vi "RFmx_Control.vi"(8 "error in (no error)":errorcluster, 10 "Device Resources":T1={"RFSG Resource in"="VST", "RFSA Resource in"="VST", "RFmx Resource in"="VST"}, 11 "Message_Queues":T2) -> (0 "error out":errorcluster)   [LabVIEW 2014]
uses:
  02_Controls/Message_Queues.ctl
  02_Controls/Message_Data_Ctl.ctl
  15_DataManagement/Device_Resources.ctl
  15_DataManagement/Config_RFmx_Settings.ctl
  <vilib>/RFmx/SpecAn/mx/RFmxSpecAn.llb/RFmxSpecAn Configure Digital Edge Trigger.vi
  <resource>/objmgr/RFmxSpecAn.rc
panel:
  out "RFSG_Msg":string
  out "Message":string
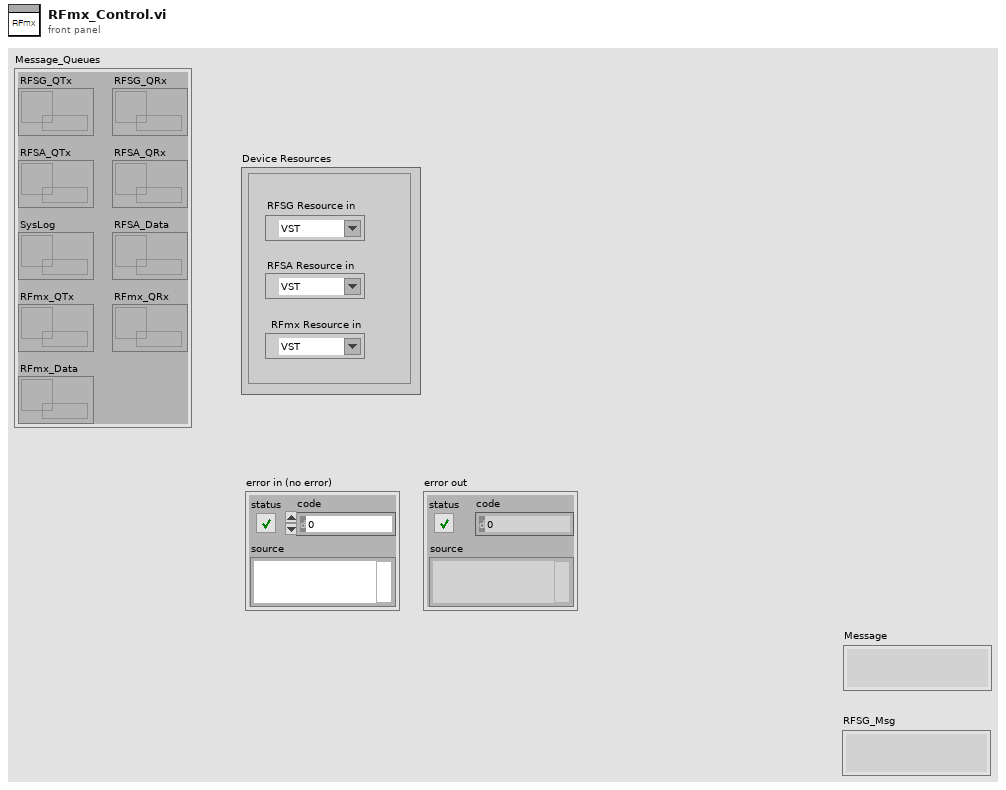
[diagram p1: front panel]
types:
  T1 = typedef "Device_Resources.ctl" = cluster{"RFSG Resource in":refnum<k15>, "RFSA Resource in":refnum<k15>, "RFmx Resource in":refnum<k15>}
  T2 = typedef "Message_Queues.ctl" = cluster{"RFSG_QTx":refnum<queue>, "RFSG_QRx":refnum<queue>, "RFSA_QTx":refnum<queue>, "RFSA_QRx":refnum<queue>, "SysLog":refnum<queue>, "RFSA_Data":refnum<queue>, "RFmx_QTx":refnum<queue>, "RFmx_QRx":refnum<queue>, "RFmx_Data":refnum<queue>}
  T3 = typedef "Config_RFmx_Settings.ctl" = cluster{"Default":cluster{"Center_Freq(Hz)":dbl, "Ref_Level(dBm)":dbl, "Span(Hz)":dbl, "RBW(Hz)":dbl, "RBW Filter Type":enum16{"FFT Based", "Gaussian", "Flat", "Synch Tuned - 4", "Synch Tuned - 5"}, "Ch_IBW(Hz)":dbl, "Sweep_Time(s)":dbl, "Num_of_Average":i32, "IQ_Bandwidth(Hz)":dbl}, "ACP_Offset_Freq":dbl[], "ACP_Offset_IBW":dbl[], "OBW_Percent(%)":dbl, "TXP_Interval(s)":dbl, "CCDF_Interval(s)":dbl, "CCDF_Threshold":dbl, "SFDR_Span(Hz)":dbl, "Harms_RBW(Hz)":dbl, "Harms_RBW_Filter":enum16{"FFT Based", "Gaussian", "Flat", "Synch Tuned - 4", "Synch Tuned - 5"}}
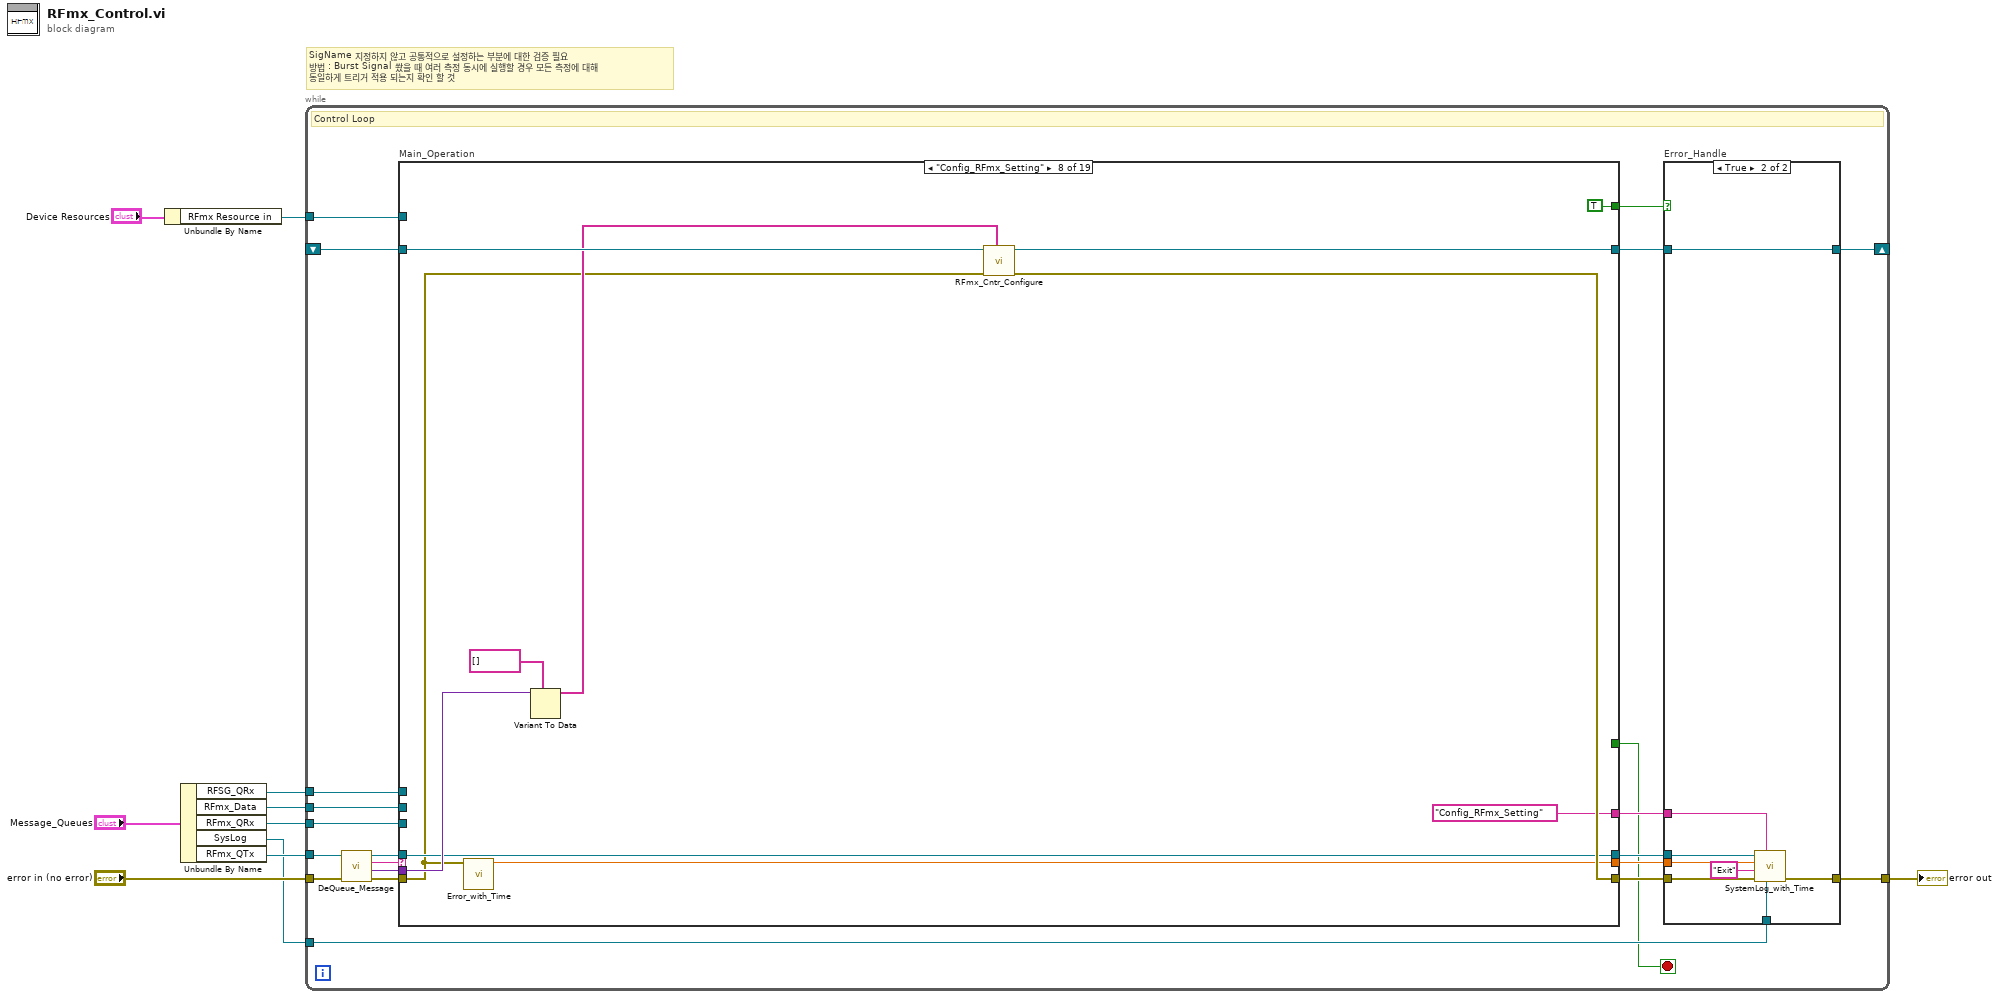
[diagram p0: block diagram]
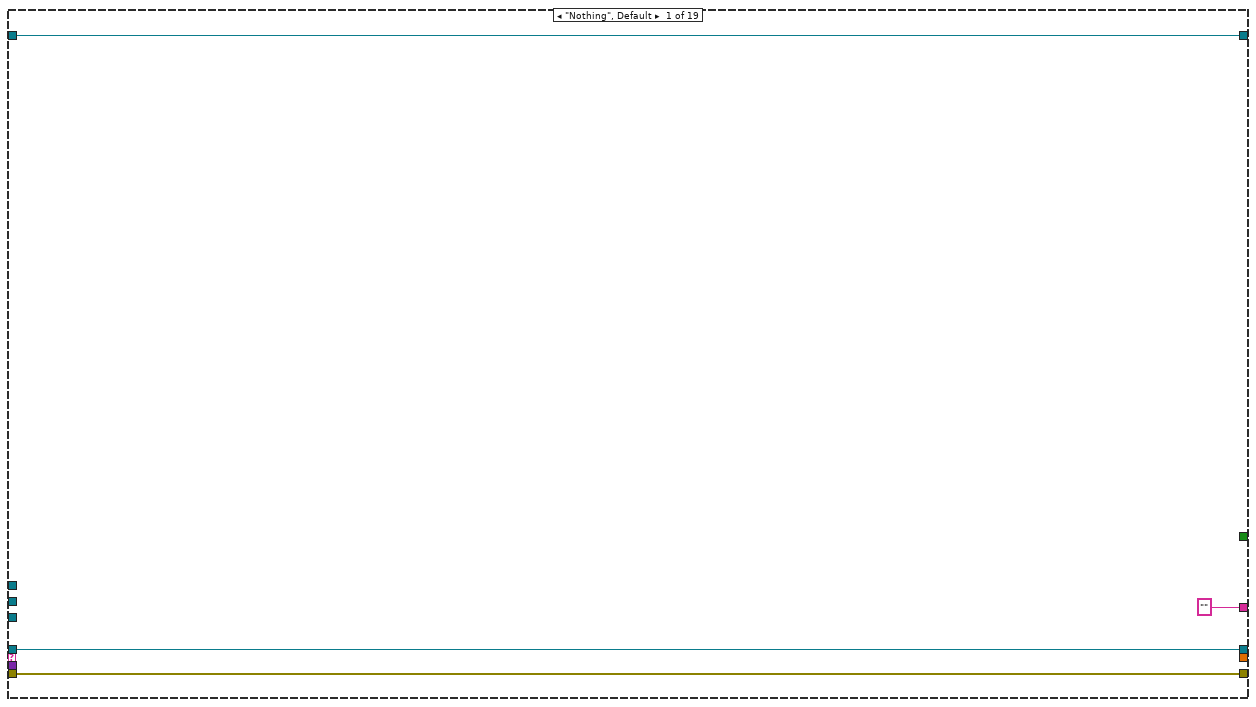
[diagram p3: hidden frame]
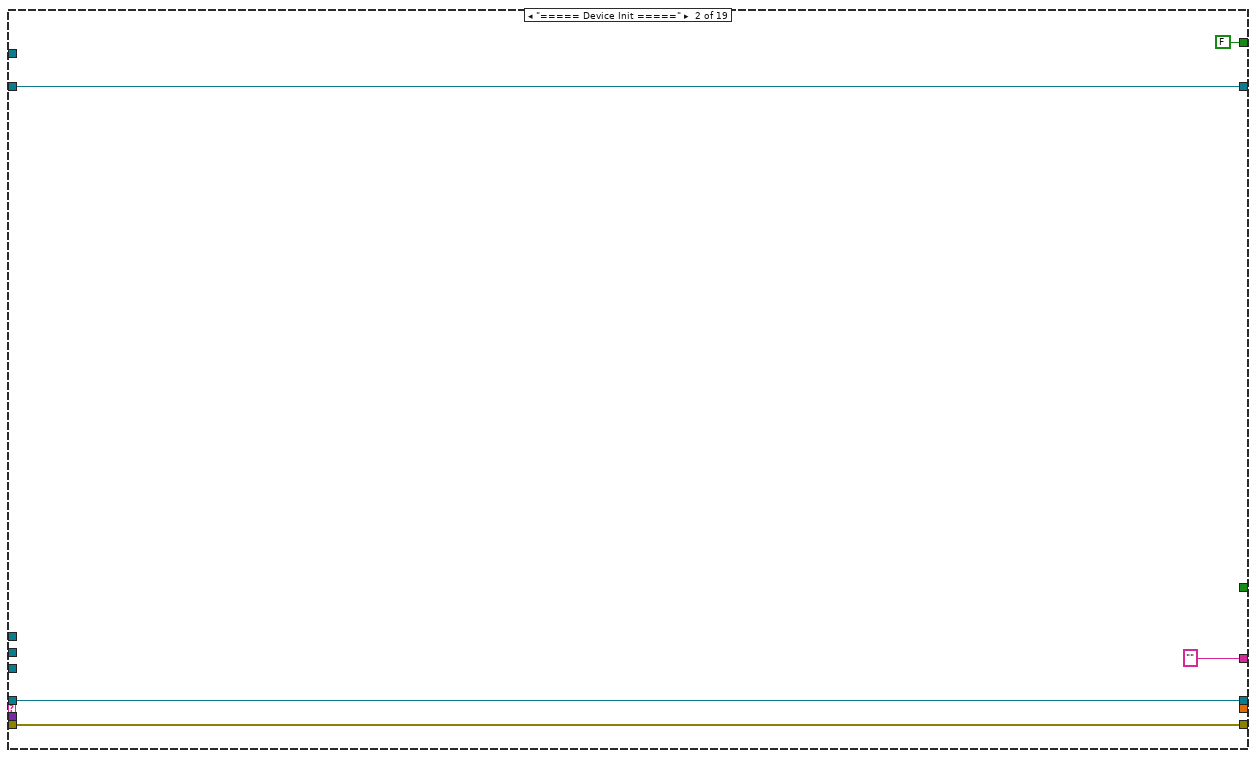
[diagram p4: hidden frame]
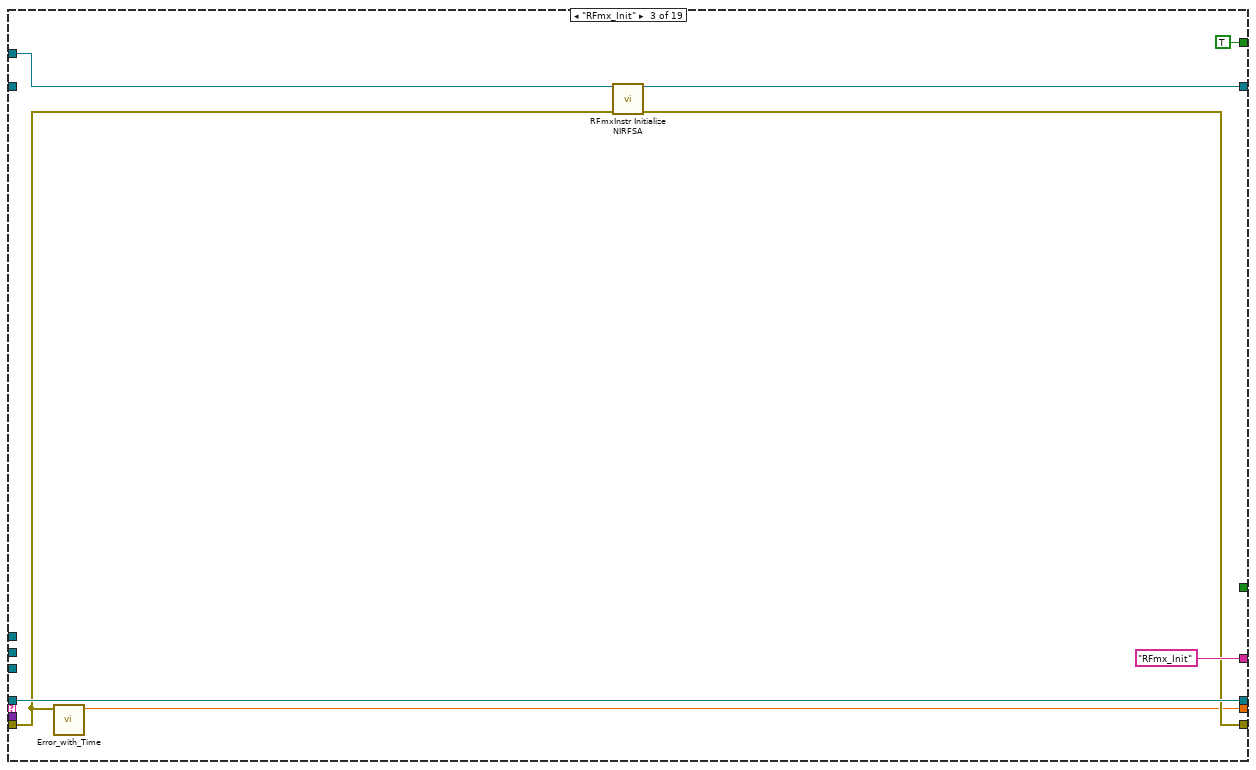
[diagram p5: hidden frame]
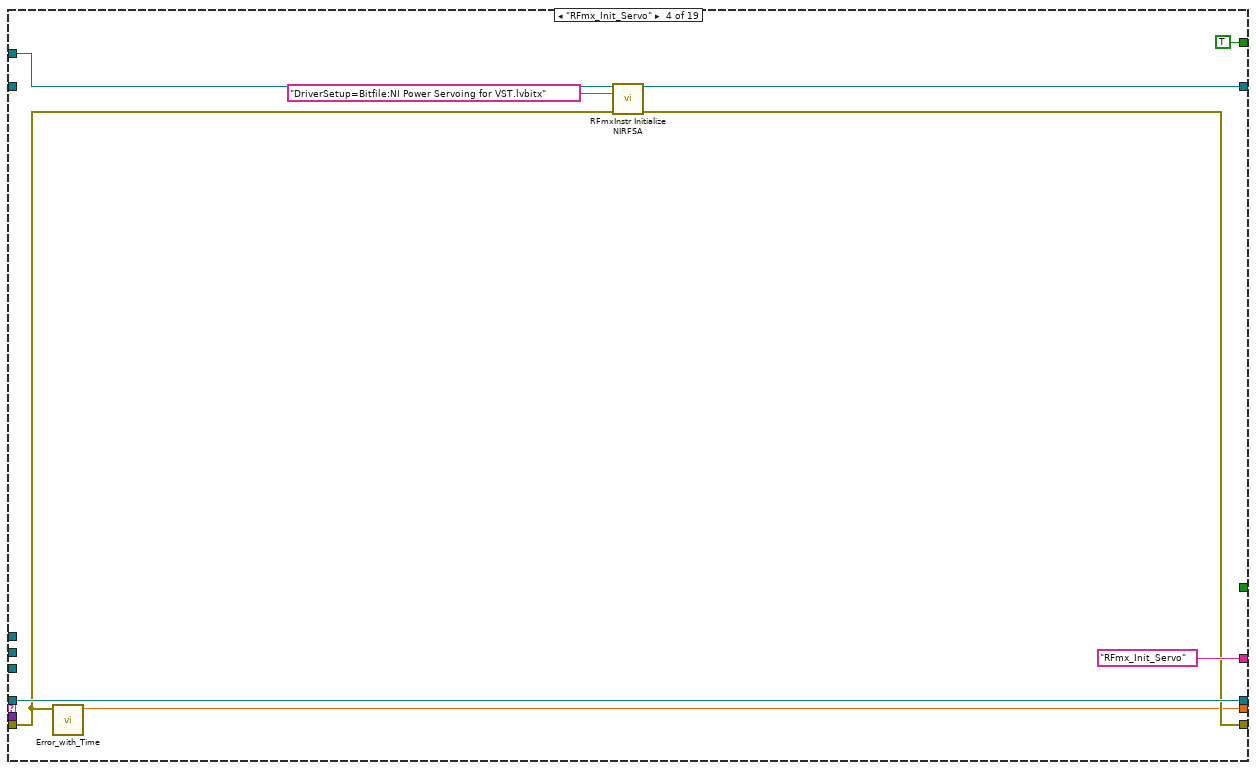
[diagram p6: hidden frame]
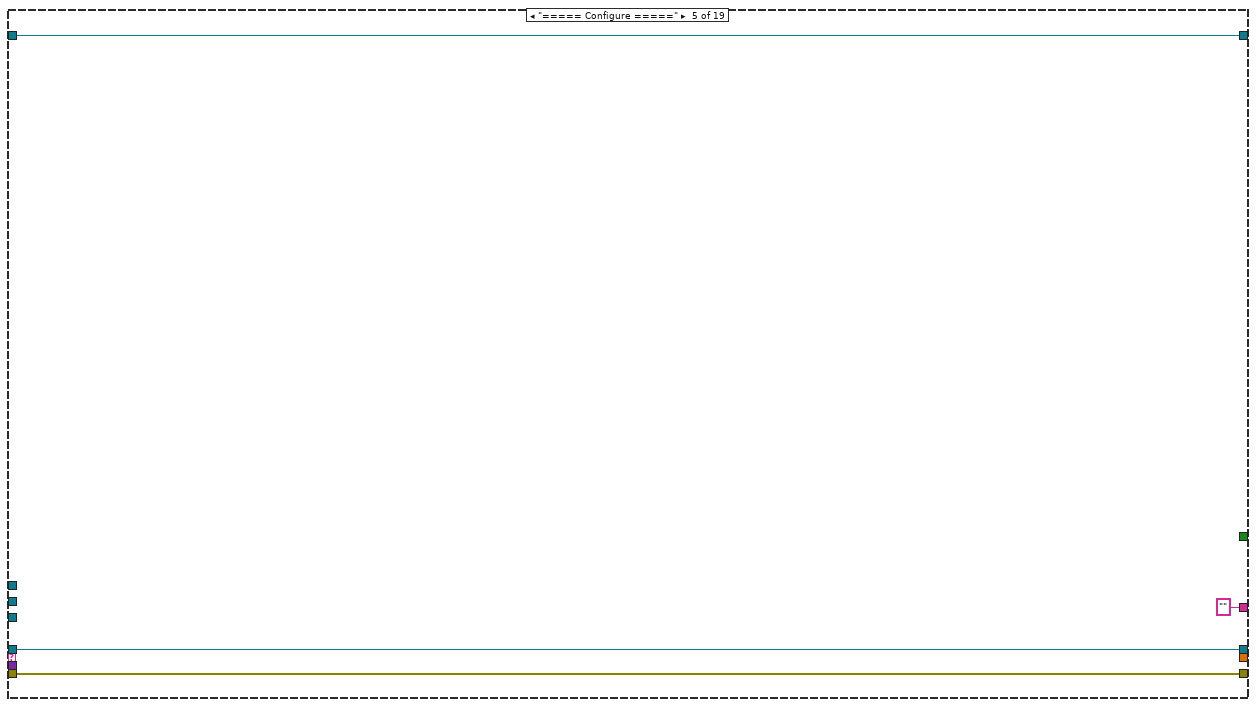
[diagram p7: hidden frame]
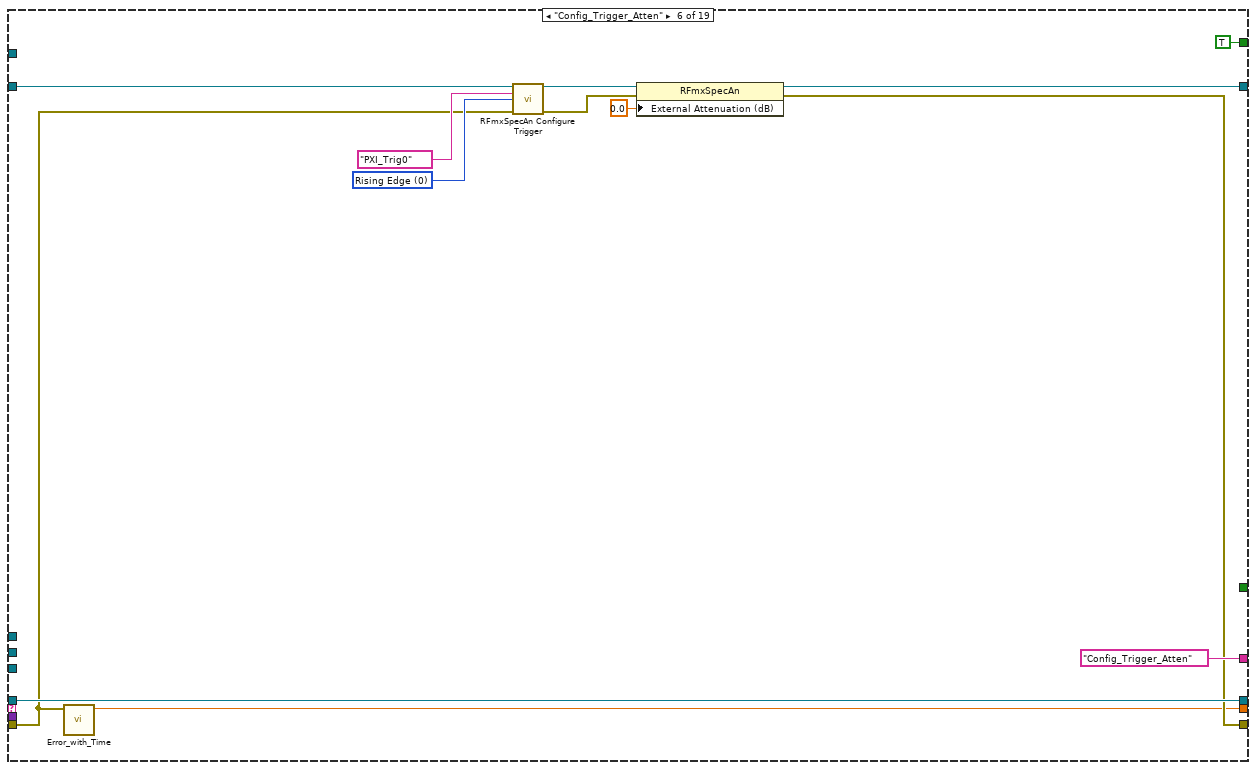
[diagram p8: hidden frame]
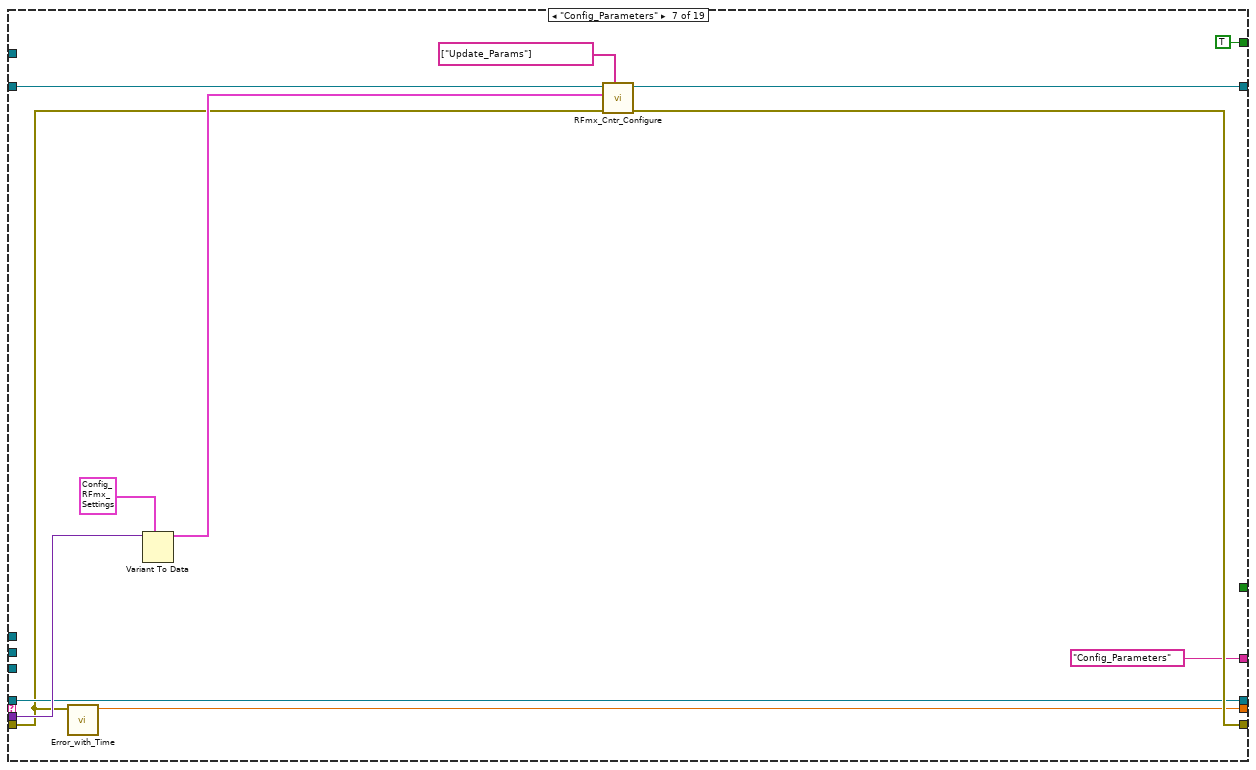
[diagram p9: hidden frame]
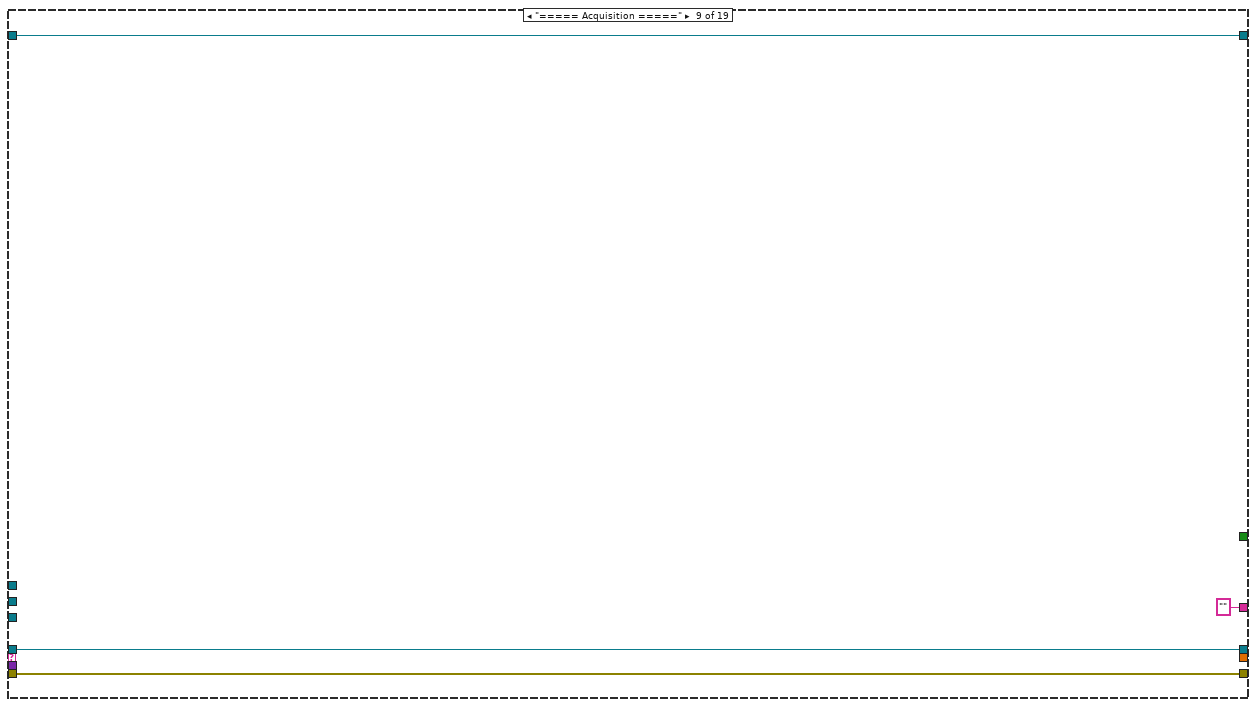
[diagram p10: hidden frame]
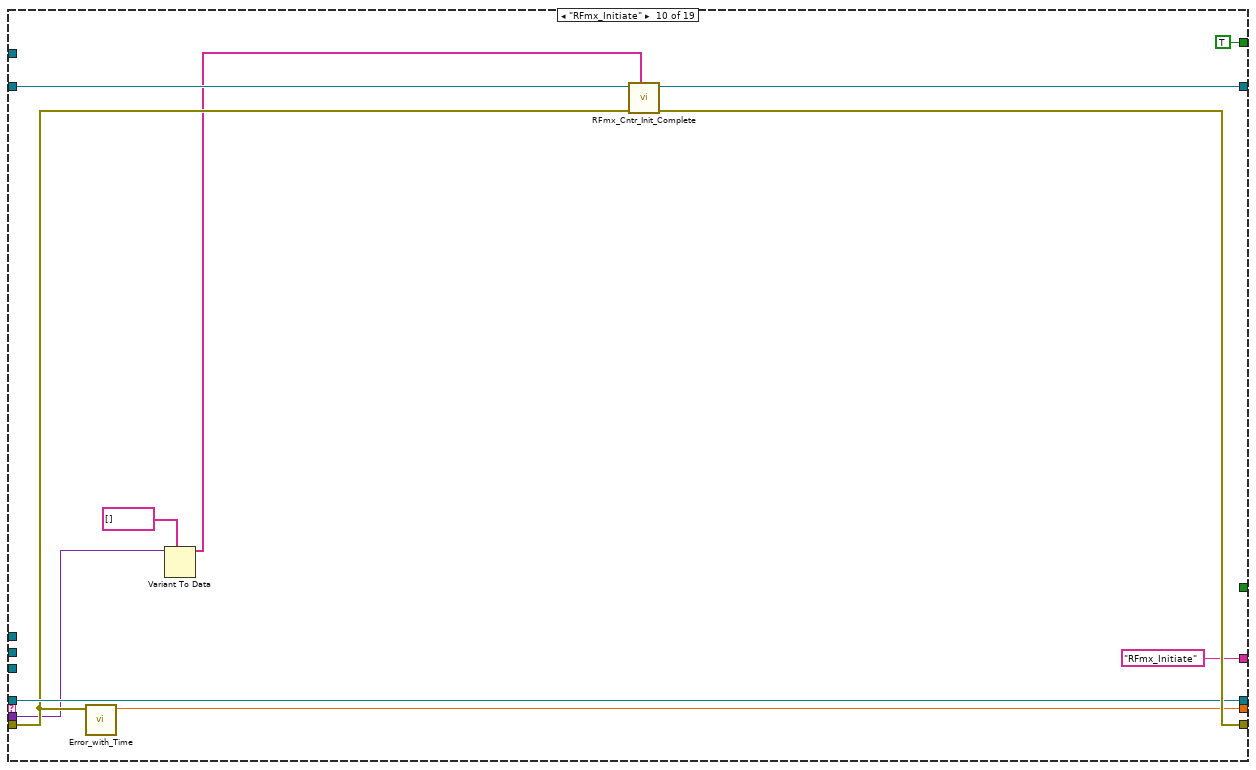
[diagram p11: hidden frame]
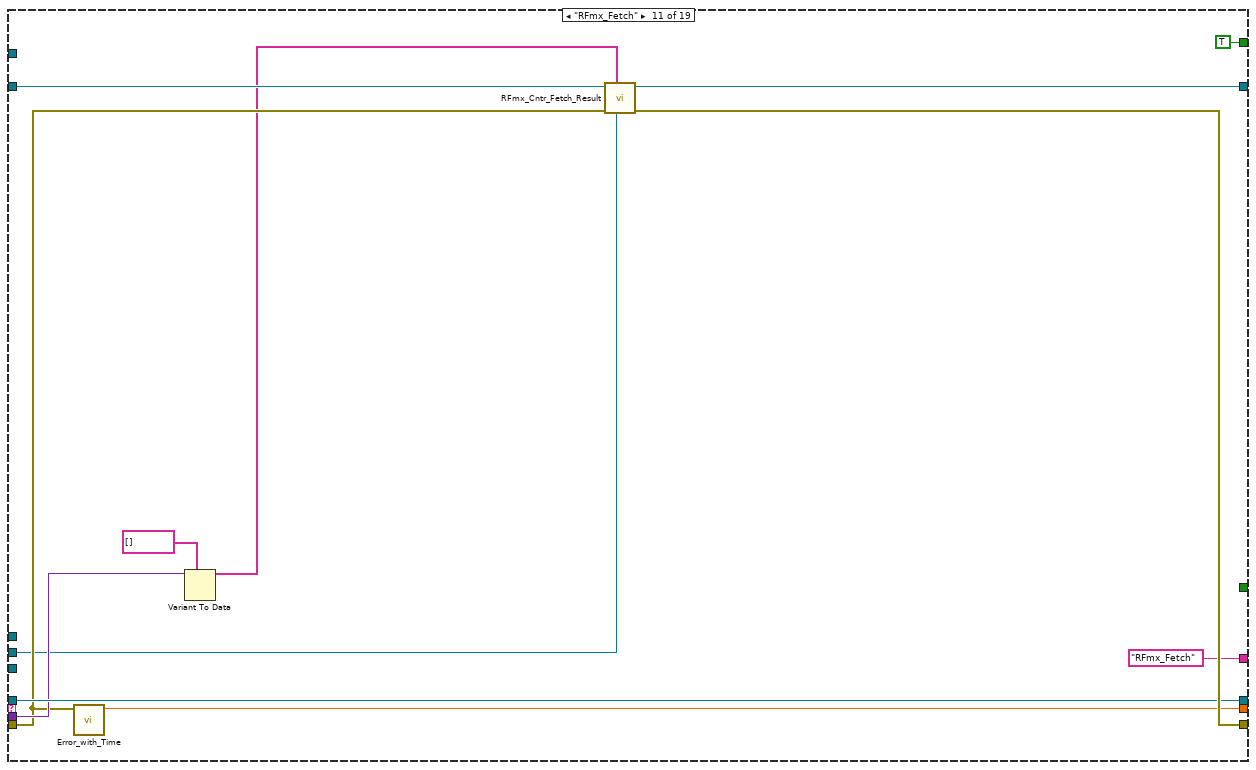
[diagram p12: hidden frame]
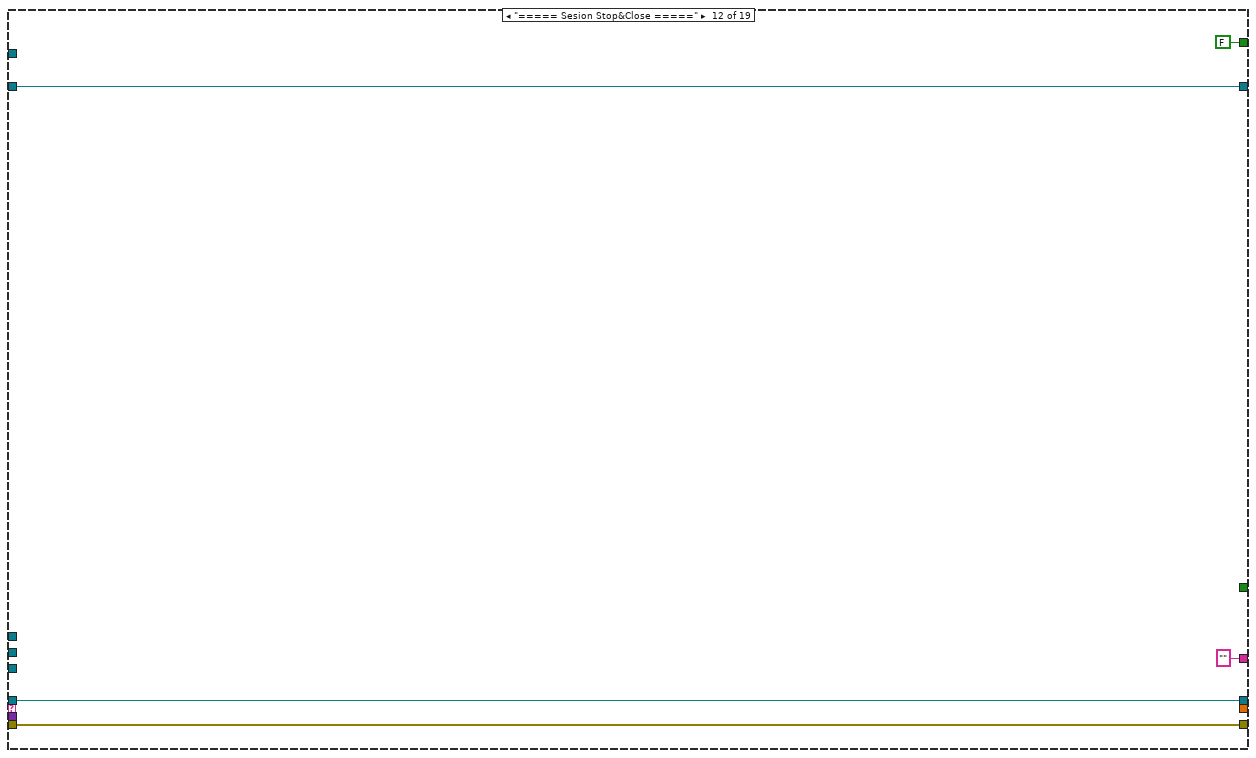
[diagram p13: hidden frame]
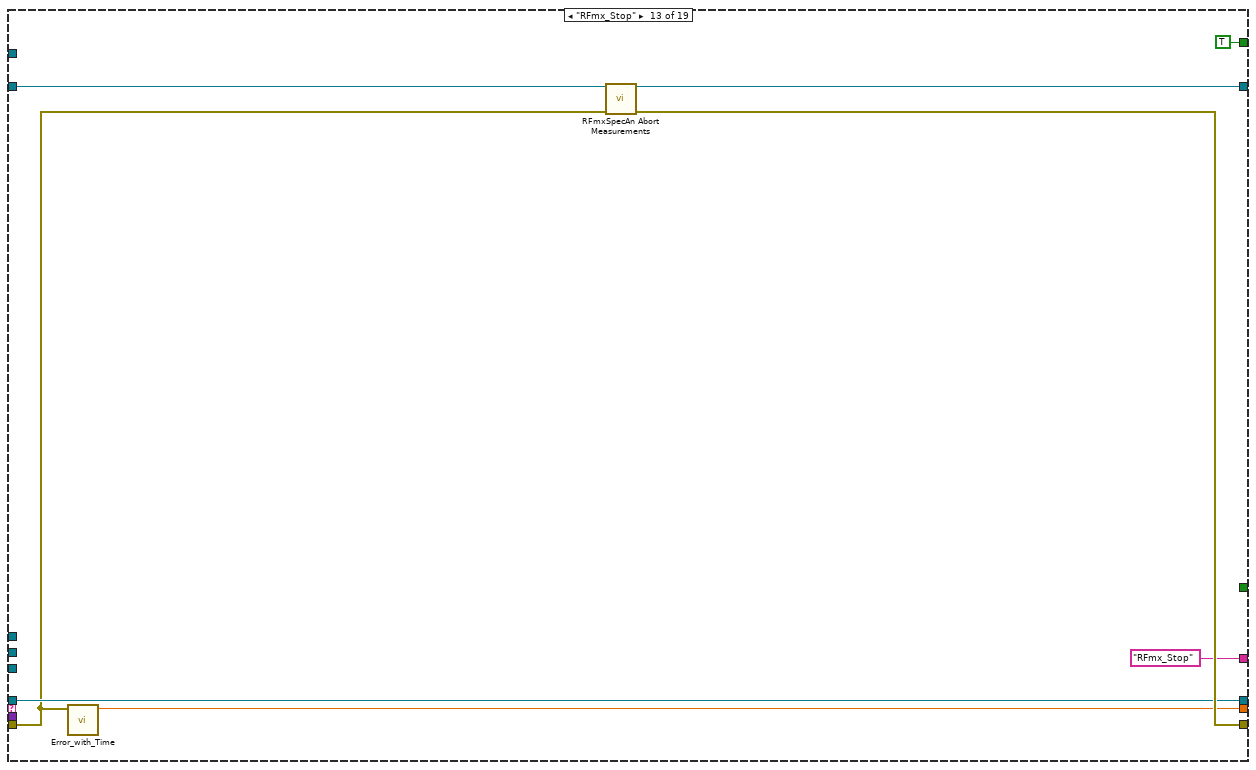
[diagram p14: hidden frame]
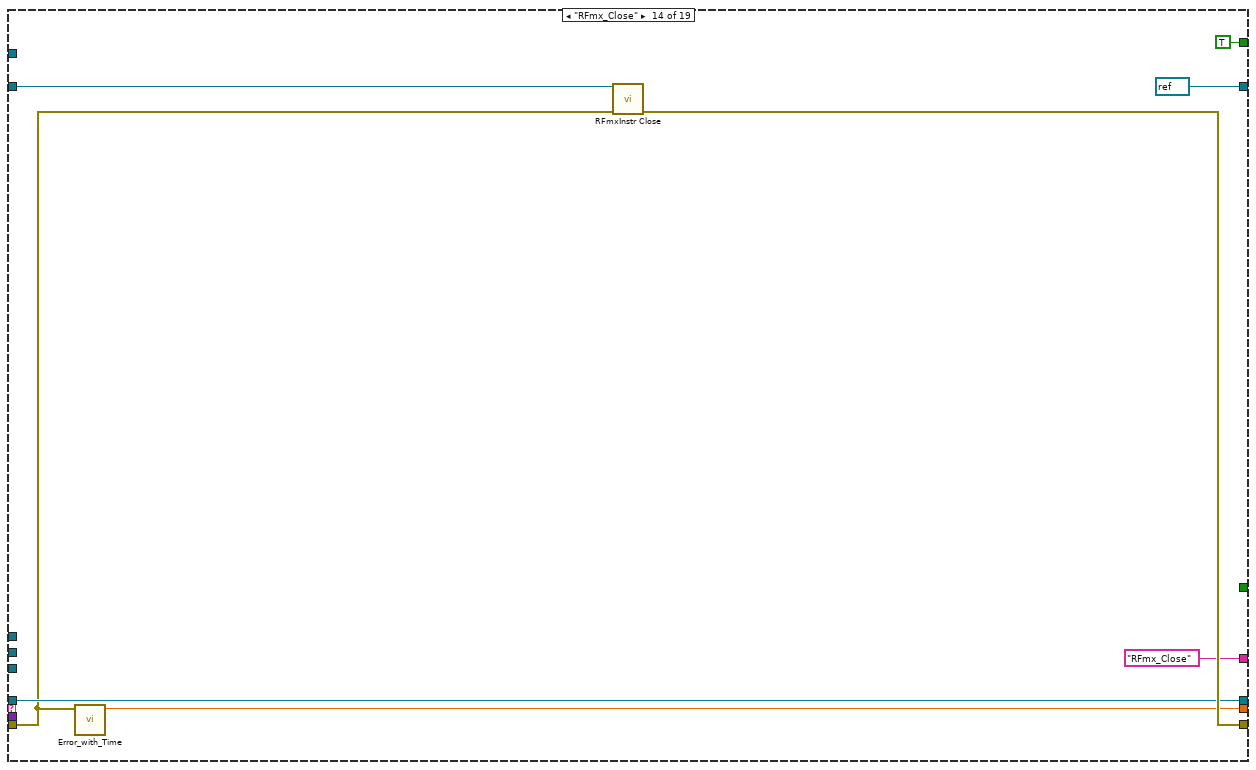
[diagram p15: hidden frame]
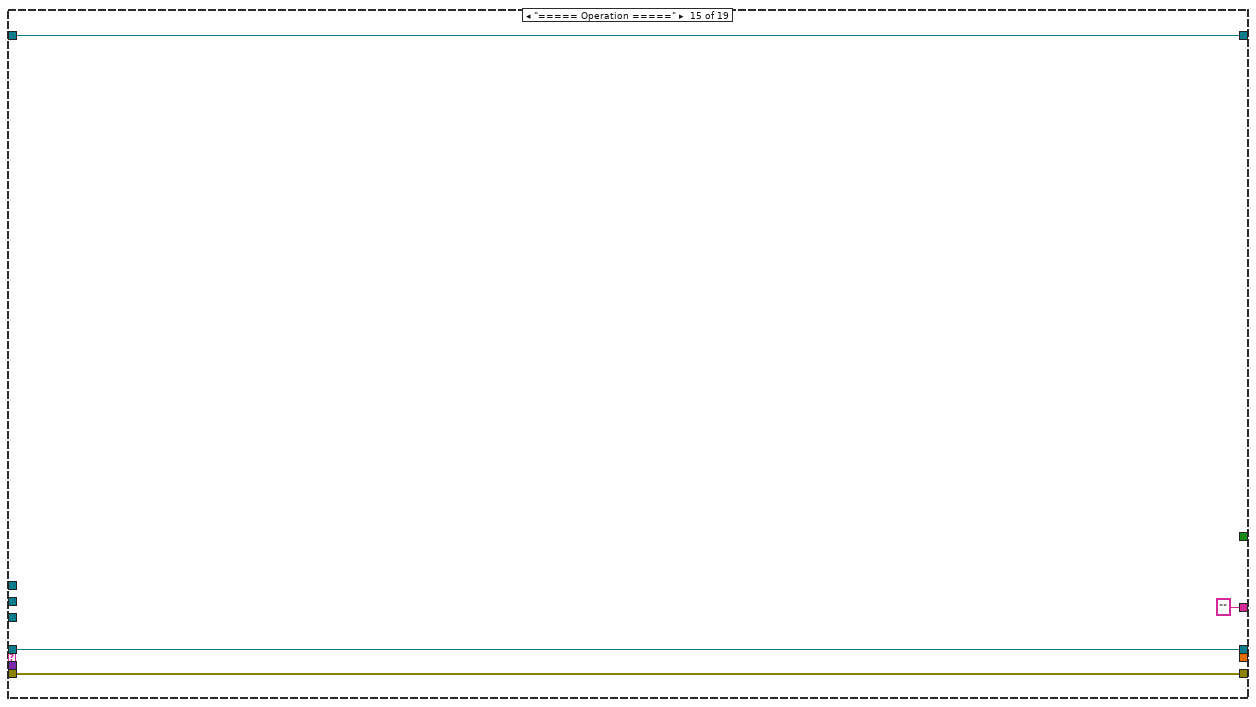
[diagram p16: hidden frame]
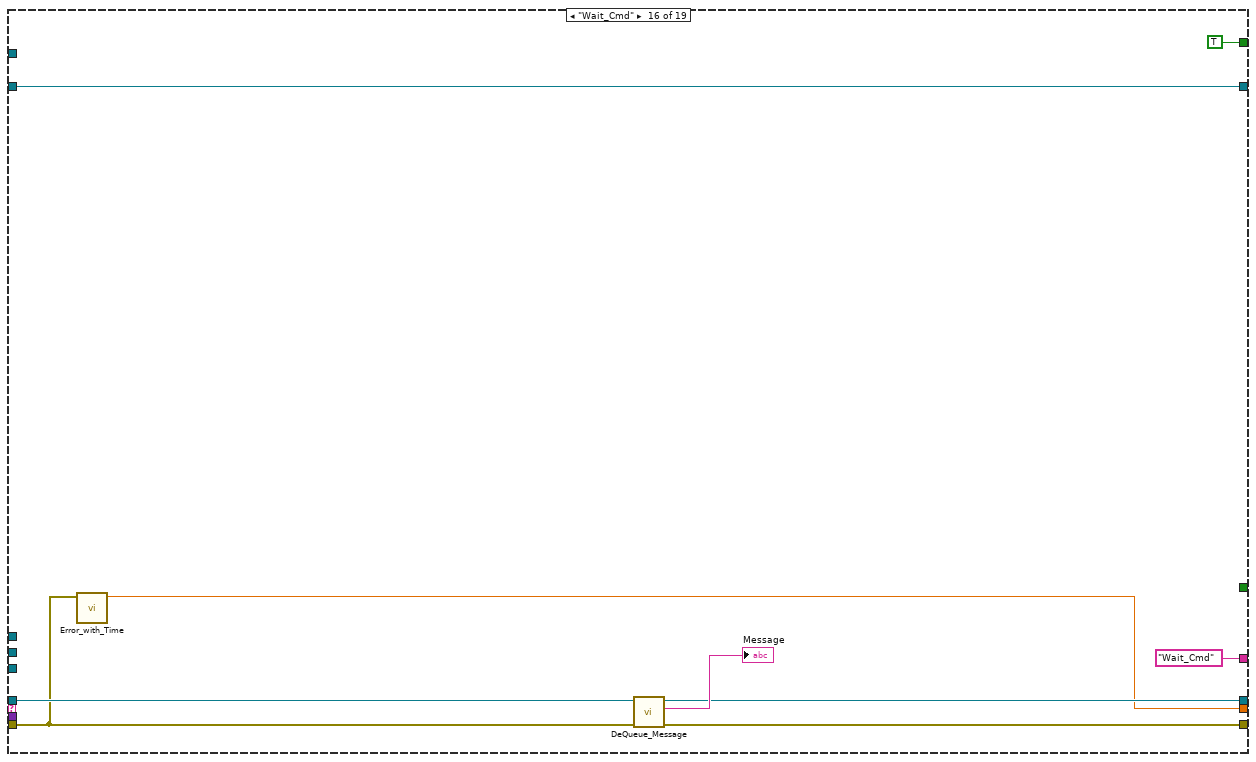
[diagram p17: hidden frame]
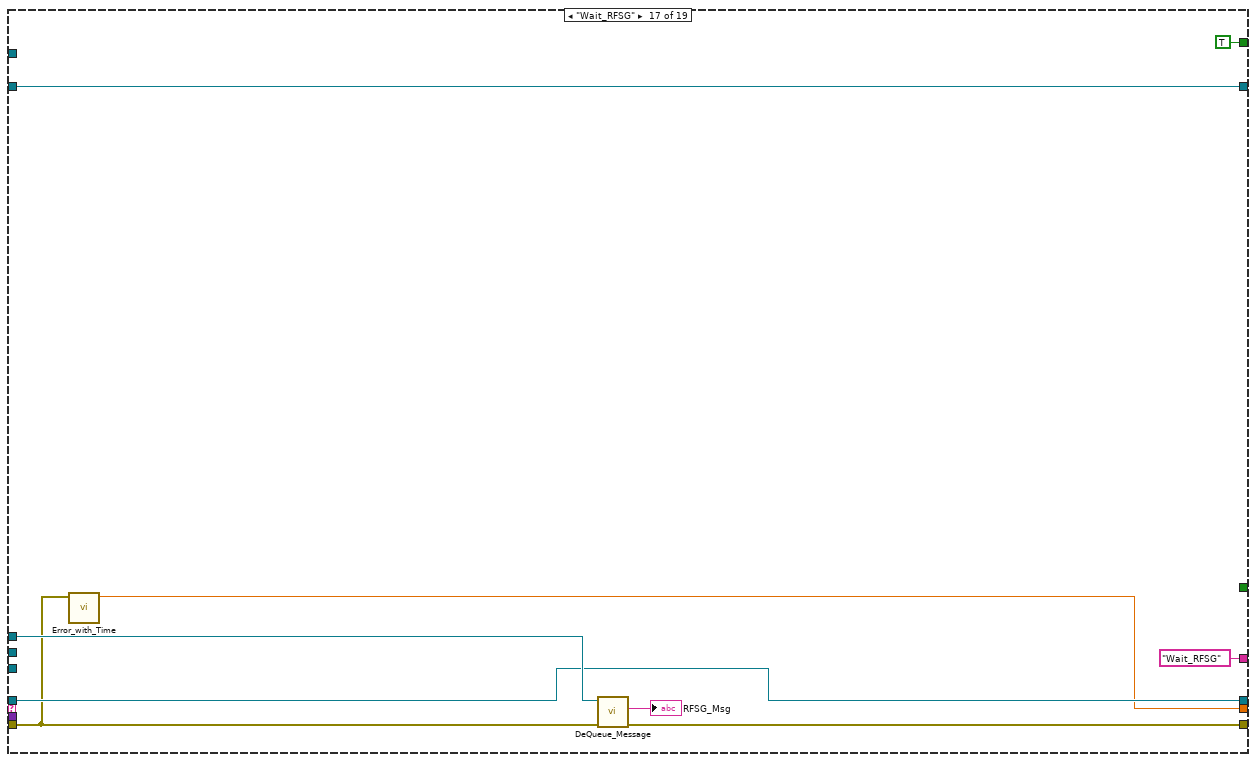
[diagram p18: hidden frame]
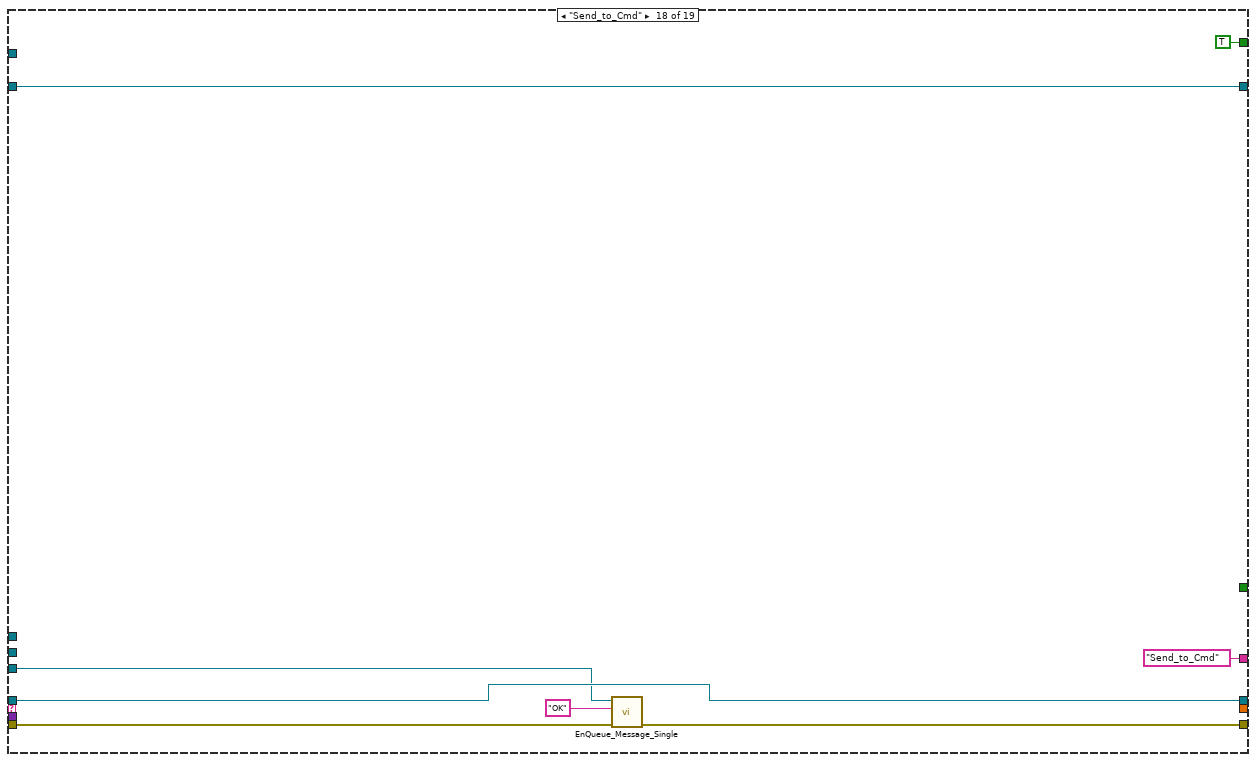
[diagram p19: hidden frame]
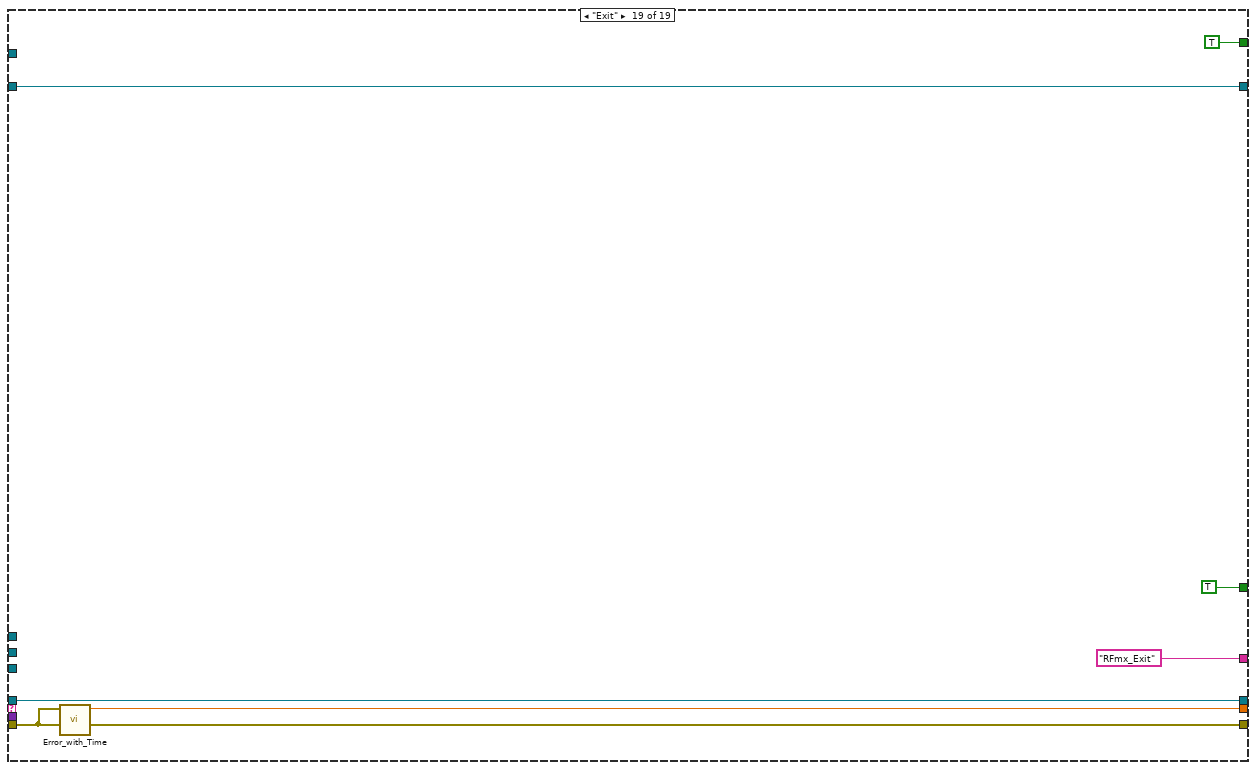
[diagram p20: hidden frame]
diagram:
  # "SigName 지정하지 않고 공통적으로 설정하는 부분에 대한 검증 필요\n방법 : Burst Signal 쐈을 때 여러 측정 동시에 실행할 경우 모든 측정에 대해\n동일하게 트리거 적용 되는지 확인 할 것"
  n1 = Unbundle By Name("Device Resources") -> ("RFmx Resource in"=w3:refnum<k15>)
  n2 = Unbundle By Name("Message_Queues") -> ("RFSG_QRx"=w1:refnum<queue>, "RFmx_Data"=w2:refnum<queue>, "RFmx_QRx"=w6:refnum<queue>, "SysLog"=w5:refnum<queue>, "RFmx_QTx"=w8:refnum<queue>)
  n3 = while {
    tunnel: "error in (no error)" -> [w31]
    tunnel: [w24] -> w9
    tunnel: w8 -> [w26]
    tunnel: w6 -> [w25]
    tunnel: w5 -> [w19]
    shift-right: [w14] -> _
    shift-left: _ -> [w16]
    tunnel: w3 -> [w13]
    tunnel: w2 -> [w12]
    tunnel: w1 -> [w11]
    stop <- w18 stop-if-true
    # "Control Loop"
    n4 = call "DeQueue_Message.vi"("error in (no error)"=w31, "Message_Queue"=w26) -> ("error out"=w27:errorcluster, "Message Data"=w29:variant, "Message"=w30:string, "Dup_Message_Queue"=w28:refnum<queue>)  [unwired: 6 in]
    n5 = case "Main_Operation" shown="\"Config_RFmx_Setting\"" w30 {
      tunnel: w29 -> [_ _ _ _ _ _ w95 w107 _ w113 w128 _ _ _ _ _ _ _ _]
      tunnel: w28 -> [w43 w49 w57 w66 w69 w82 w90 w103 w110 w118 w130 w137 w143 w152 w158 w166 w173 w181 w190]
      tunnel: w27 -> [w45 w46 w52 w61 w70 w73 w85 w98 w109 w117 w127 w136 w142 w150 w157 w163 w172 w183 w187]
      tunnel: [_ _ _ _ _ _ _ _ _ _ _ _ _ _ _ _ _ _ TRUE] -> w18
      tunnel: [w45 w46 w54 w63 w70 w76 w91 w104 w109 w120 w132 w136 w145 w154 w157 w164 w175 w182 w187] -> w22
      tunnel: w25 -> [_ _ _ _ _ _ _ _ _ _ _ _ _ _ _ _ _ w180 _]
      tunnel: ["" ("Message") "" ("Message") "RFmx_Init" ("Message") "RFmx_Init_Servo" ("Message") "" ("Message") "Config_Trigger_Atten" ("Message") "Config_Parameters" ("Message") "Config_RFmx_Setting" ("Message") "" ("Message") "RFmx_Initiate" ("Message") "RFmx_Fetch" ("Message") "" ("Message") "RFmx_Stop" ("Message") "RFmx_Close" ("Message") "" ("Message") "Wait_Cmd" ("Message") "Wait_RFSG" ("Message") "Send_to_Cmd" ("Message") "RFmx_Exit" ("Message")] -> w23
      tunnel: [_ _ w51 w60 _ w74 w86 w97 _ w116 w126 _ w141 w151 _ w162 w171 _ w188] -> w21
      tunnel: [w43 w49 w57 w66 w69 w82 w90 w103 w110 w118 w130 w137 w143 w152 w158 w165 w173 w181 w190] -> w20
      tunnel: [_ FALSE TRUE TRUE _ TRUE TRUE TRUE _ TRUE TRUE FALSE TRUE TRUE _ TRUE TRUE TRUE TRUE] -> w17
      tunnel: [w42 w47 w56 w65 w71 w77 w93 w105 w111 w121 w133 w139 w146 refnum<k21> refnum ("Instrument Handle Out") w159 w168 w177 w185 w186] -> w15
      tunnel: w16 -> [w42 w47 _ _ w71 w83 w94 w106 w111 w122 w134 w139 w147 w155 w159 w168 w177 w185 w186]
      tunnel: w13 -> [_ _ w55 w64 _ _ _ _ _ _ _ _ _ _ _ _ _ _ _]
      tunnel: w12 -> [_ _ _ _ _ _ _ _ _ _ w123 _ _ _ _ _ _ _ _]
      tunnel: w11 -> [_ _ _ _ _ _ _ _ _ _ _ _ _ _ _ _ w174 _ _]
      frame "Nothing", Default {
      }
      frame "===== Device Init =====" {
      }
      frame "RFmx_Init" {
        n6 = call "Error_with_Time.vi"("error in (no error)"=w52) -> ("relative seconds"=w51:dbl)  [unwired: 10 in]
        n7 = call <vilib>:"RFmxInstr Initialize NIRFSA.vi"("Resource Name"=w55, "error in (no error)"=w52) -> ("Instrument Handle Out"=w56:refnum<k21>, "error out"=w54:errorcluster)  [unwired: 11 in, 1 out]
      }
      frame "RFmx_Init_Servo" {
        n8 = call "Error_with_Time.vi"("error in (no error)"=w61) -> ("relative seconds"=w60:dbl)  [unwired: 10 in]
        n9 = call <vilib>:"RFmxInstr Initialize NIRFSA.vi"("Resource Name"=w64, "Option String"="DriverSetup=Bitfile:NI Power Servoing for VST.lvbitx" ("Bitfile"), "error in (no error)"=w61) -> ("Instrument Handle Out"=w65:refnum<k21>, "error out"=w63:errorcluster)  [unwired: 10 in, 1 out]
      }
      frame "===== Configure =====" {
      }
      frame "Config_Trigger_Atten" {
        w80 = 0 items=["Rising Edge", "Falling Edge"] ("Digital Edge")
        n10 = call "Error_with_Time.vi"("error in (no error)"=w73) -> ("relative seconds"=w74:dbl)  [unwired: 10 in]
        n11 = call-poly <vilib>:"RFmxSpecAn Configure Trigger.vi"("Instrument Handle In"=w83, "Digital Edge Source"="PXI_Trig0", "Digital Edge"=w80, "error in (no error)"=w73) -> ("Instrument Handle Out"=w79:refnum<k21>, "error out"=w78:errorcluster)  [unwired: 10 in]
        n12 = property class="RFmxSpecAn"(reference=w79, error in=w78, "External Attenuation (dB)"=0.0) -> (reference out=w77:refnum<k21>, error out=w76:errorcluster)
      }
      frame "Config_Parameters" {
        n13 = call "Error_with_Time.vi"("error in (no error)"=w85) -> ("relative seconds"=w86:dbl)  [unwired: 10 in]
        n14 = Variant To Data(type=T3 {"Default"={"Center_Freq(Hz)"=1150000000.0, "Ref_Level(dBm)"=-10.0, "Span(Hz)"=20000000.0, "RBW(Hz)"=10000.0, "RBW Filter Type"=enum."Gaussian", "Ch_IBW(Hz)"=3840000.0, "Sweep_Time(s)"=0.01, "Num_of_Average"=10, "IQ_Bandwidth(Hz)"=20000000.0}, "ACP_Offset_Freq"=[5000000.0, 10000000.0, 12500000.0], "ACP_Offset_IBW"=[3840000.0, 3840000.0, 3840000.0], "OBW_Percent(%)"=95.0, "TXP_Interval(s)"=0.01, "CCDF_Interval(s)"=0.01, "CCDF_Threshold"=-30.0, "SFDR_Span(Hz)"=20000000.0, "Harms_RBW(Hz)"=10000.0, "Harms_RBW_Filter"=enum."Gaussian"} ("RFmx_Parameters"), Variant=w95) -> (data=w92:T3)  [unwired: 1 in, 1 out]
        n15 = call "RFmx_Cntr_Configure.vi"("Meas_Type"=string[] ["Update_Params"], "error in (no error)"=w85, "RFmx_Parameters"=w92, "Instrument Handle in"=w94) -> ("error out"=w91:errorcluster, "Instrument Handle out"=w93:refnum<k21>)  [unwired: 6 in]
      }
      frame "Config_RFmx_Setting" {
        n16 = call "Error_with_Time.vi"("error in (no error)"=w98) -> ("relative seconds"=w97:dbl)  [unwired: 10 in]
        n17 = Variant To Data(type=string[] [], Variant=w107) -> (data=w99:string[])  [unwired: 1 in, 1 out]
        n18 = call "RFmx_Cntr_Configure.vi"("Meas_Type"=w99, "error in (no error)"=w98, "Instrument Handle in"=w106) -> ("error out"=w104:errorcluster, "Instrument Handle out"=w105:refnum<k21>)  [unwired: 7 in]
      }
      frame "===== Acquisition =====" {
      }
      frame "RFmx_Initiate" {
        n19 = call "Error_with_Time.vi"("error in (no error)"=w117) -> ("relative seconds"=w116:dbl)  [unwired: 10 in]
        n20 = Variant To Data(type=string[] [], Variant=w113) -> (data=w112:string[])  [unwired: 1 in, 1 out]
        n21 = call "RFmx_Cntr_Init_Complete.vi"("Meas_Type"=w112, "error in (no error)"=w117, "Instrument Handle in"=w122) -> ("error out"=w120:errorcluster, "Instrument Handle out"=w121:refnum<k21>)  [unwired: 7 in]
      }
      frame "RFmx_Fetch" {
        n22 = call "Error_with_Time.vi"("error in (no error)"=w127) -> ("relative seconds"=w126:dbl)  [unwired: 10 in]
        n23 = Variant To Data(type=string[] [], Variant=w128) -> (data=w125:string[])  [unwired: 1 in, 1 out]
        n24 = call "RFmx_Cntr_Fetch_Result.vi"("RFmx_Data_In"=w123, "Meas_Type"=w125, "error in (no error)"=w127, "Instrument Handle in"=w134) -> ("error out"=w132:errorcluster, "Instrument Handle out"=w133:refnum<k21>)  [unwired: 6 in]
      }
      frame "===== Sesion Stop&Close =====" {
      }
      frame "RFmx_Stop" {
        n25 = call "Error_with_Time.vi"("error in (no error)"=w142) -> ("relative seconds"=w141:dbl)  [unwired: 10 in]
        n26 = call <vilib>:"RFmxSpecAn Abort Measurements.vi"("Instrument Handle In"=w147, "error in (no error)"=w142) -> ("Instrument Handle Out"=w146:refnum<k21>, "error out"=w145:errorcluster)  [unwired: 12 in]
      }
      frame "RFmx_Close" {
        n27 = call "Error_with_Time.vi"("error in (no error)"=w150) -> ("relative seconds"=w151:dbl)  [unwired: 10 in]
        n28 = call <vilib>:"RFmxInstr Close.vi"("Instrument Handle In"=w155, "error in (no error)"=w150) -> ("error out"=w154:errorcluster)  [unwired: 13 in]
      }
      frame "===== Operation =====" {
      }
      frame "Wait_Cmd" {
        n29 = call "Error_with_Time.vi"("error in (no error)"=w163) -> ("relative seconds"=w162:dbl)  [unwired: 10 in]
        n30 = call "DeQueue_Message.vi"("error in (no error)"=w163, "Message_Queue"=w166) -> ("error out"=w164:errorcluster, "Message"=→"Message":string, "Dup_Message_Queue"=w165:refnum<queue>)  [unwired: 6 in, 1 out]
      }
      frame "Wait_RFSG" {
        n31 = call "Error_with_Time.vi"("error in (no error)"=w172) -> ("relative seconds"=w171:dbl)  [unwired: 10 in]
        n32 = call "DeQueue_Message.vi"("error in (no error)"=w172, "Message_Queue"=w174) -> ("error out"=w175:errorcluster, "Message"=→"RFSG_Msg":string)  [unwired: 6 in, 2 out]
      }
      frame "Send_to_Cmd" {
        n33 = call "EnQueue_Message_Single.vi"("error in (no error)"=w183, "Message"="OK", "Message_Queue"=w180) -> ("error out"=w182:errorcluster)  [unwired: 7 in, 1 out]
      }
      frame "Exit" {
        n34 = call "Error_with_Time.vi"("error in (no error)"=w187) -> ("relative seconds"=w188:dbl)  [unwired: 10 in]
      }
    }
    n35 = case "Error_Handle" shown="True" w17 {
      tunnel: w22 -> [w33 w41]
      tunnel: [w33 w40] -> w24
      tunnel: w23 -> [_ w39]
      tunnel: w20 -> [_ w38]
      tunnel: w21 -> [_ w37]
      tunnel: w19 -> [_ w36]
      tunnel: w15 -> [w32 w34]
      tunnel: [w32 w34] -> w14
      frame False {
      }
      frame True {
        n36 = call "SystemLog_with_Time.vi"("SysLog_Queue"=w36, "Message_in"=w39, "error in (no error)"=w41, "Send_Msg"="Exit", "Tick_in"=w37, "Worker_Queue"=w38) -> ("error out"=w40:errorcluster)  [unwired: 5 in]
      }
    }
  }
  "error out" <- w9
